vi "Get Max Level.vi"(8 "error in (no error)":errorcluster, 10 "Name":string, 11 "SignalManager in":refnum<class "SignalManager.lvclass">) -> (0 "error out":errorcluster, 2 "Max level":dbl, 3 "SignalManager out":refnum<class "SignalManager.lvclass">)   [LabVIEW 2020, in "SignalManager.lvclass"]
uses:
  SignalManager.lvclass
  SignalManager.lvclass/SignalManager.ctl
  Channel/Channel.lvclass/Channel.ctl
  Level/Level.lvclass/Level.ctl
  Channel/Read Level.vi
  Channel/Read Name.vi
  Level/Read max.vi
  Level/Level.lvclass
  Channel/Channel.lvclass
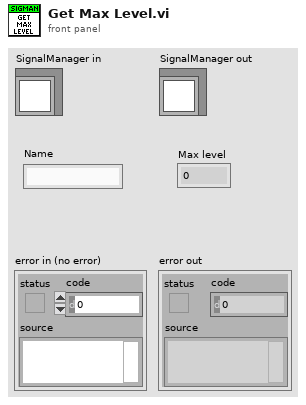
[diagram p1: front panel]
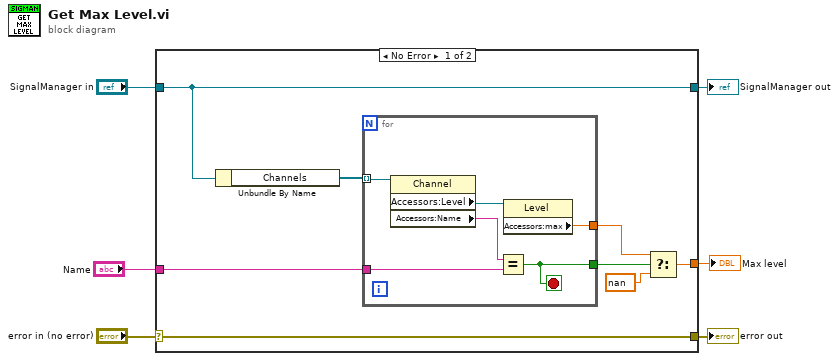
[diagram p0: block diagram]
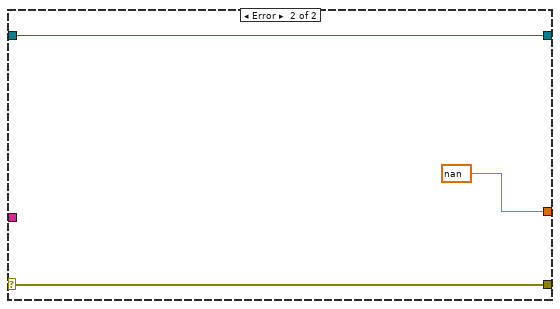
[diagram p2: hidden frame]
diagram:
  n1 = case shown="No Error" "error in (no error)" {
    selector: "error in (no error)" -> [w14 w23]
    tunnel: [w14 w23] -> w5
    tunnel: [w13 w22] -> w3
    tunnel: "SignalManager in" -> [w13 w22]
    tunnel: "Name" -> [w11 _]
    tunnel: [w8 nan ("Accessors:max")] -> w1
    frame No Error {
      n2 = Unbundle By Name(w13) -> ("Channels"=w12:refnum<class "Channel.lvclass">[])
      n3 = for {
        tunnel: w12 -> [w20] mode=indexing
        tunnel: [w18] -> w9
        tunnel: w11 -> [w16]
        tunnel: [w15] -> w10
        stop <- w15 stop-if-true
        n4 = property class="Channel"(reference=w20) -> ("Accessors:Level"=w19:refnum<class "Level.lvclass">, "Accessors:Name"=w17:string)  [unwired: 1 in, 2 out]
        n5 = Equal?(x=w17, y=w16) -> (x = y?=w15:bool)
        n6 = property class="Level"(reference=w19) -> ("Accessors:max"=w18:dbl)  [unwired: 1 in, 2 out]
      }
      n7 = Select(t=w9, s=w10, f=nan) -> (s? t:f=w8:dbl)
    }
    frame Error {
    }
  }
  "error out" <- w5
  "SignalManager out" <- w3
  "Max level" <- w1
